vi "ReplaceControlByLabelText.vi"(8 "error in (no error)":errorcluster, 9 "Replacement Path":path, 10 "Control Label.text":string, 11 "VI ref":refnum<vi>) -> (0 "error out":errorcluster, 2 "New Control Ref":refnum<vi>, 3 "VI ref":refnum<vi>)   [LabVIEW 2019, in "BlueUtilityScripts.lvlib"]
uses:
  BlueUtilityScripts.lvlib
  <vilib>/Utility/error.llb/Error Cluster From Error Code.vi
  <vilib>/ErrorRing/Error Ring.xnode
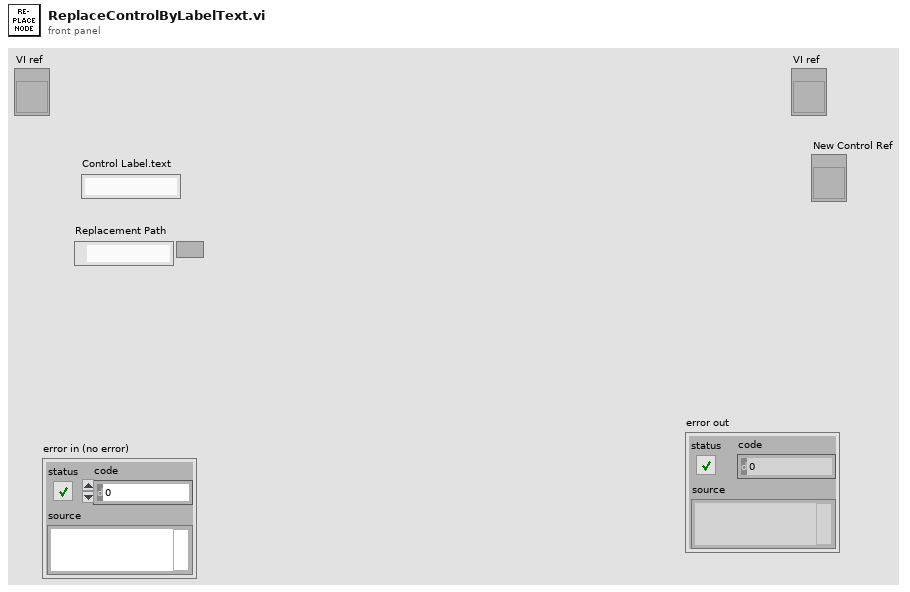
[diagram p1: front panel]
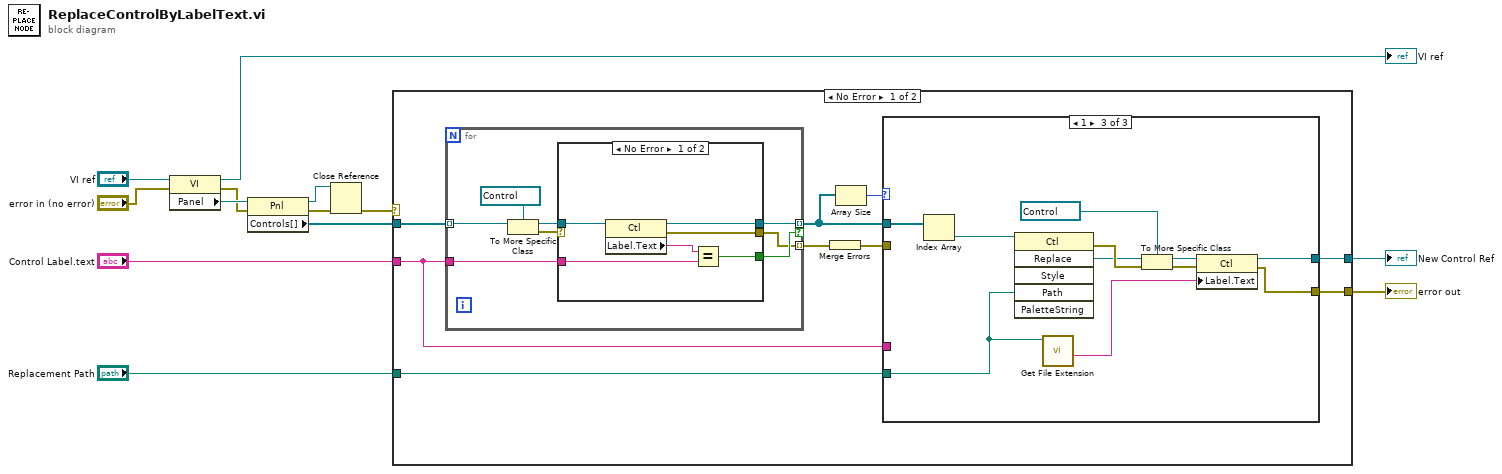
[diagram p0: block diagram]
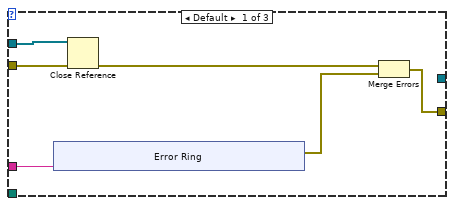
[diagram p2: hidden frame]
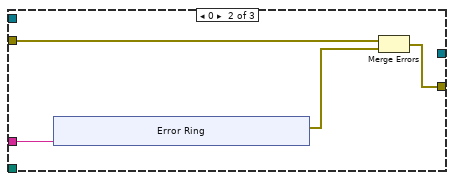
[diagram p3: hidden frame]
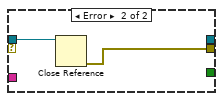
[diagram p4: hidden frame]
diagram:
  n1 = property class="VI"(reference="VI ref", error in="error in (no error)") -> (reference out=→"VI ref":refnum<vi>, error out=w8:errorcluster, "Panel"=w13:refnum<vi>)
  n2 = property class="Pnl"(reference=w13, error in=w8) -> (reference out=w6:refnum<vi>, error out=w7:errorcluster, "Controls[]"=w9:refnum<vi>[])
  n3 = Close Reference(reference=w6, error in (no error)=w7) -> (error out=w5:errorcluster)
  n4 = case shown="No Error" w5 {
    selector: w5 -> [_ w74]
    tunnel: w9 -> [w22 _]
    tunnel: "Control Label.text" -> [w20 _]
    tunnel: "Replacement Path" -> [w16 _]
    tunnel: [w15 w74] -> w1
    tunnel: [w14 _] -> w2
    frame No Error {
      n5 = for {
        tunnel: w22 -> [w65] mode=indexing
        tunnel: [w63] -> w17 mode=indexing if=w59
        tunnel: w20 -> [w60]
        tunnel: [w58] -> w19 mode=indexing
        n6 = To More Specific Class(target class=refnum<vi> refnum ("Other Refnum"), reference=w65) -> (specific class reference=w64:refnum<vi>, error out=w61:errorcluster)  [unwired: 1 in]
        n7 = case shown="No Error" w61 {
          tunnel: w64 -> [w71 w73]
          tunnel: [w70 _] -> w63
          tunnel: w60 -> [w68 _]
          tunnel: [w67 _] -> w59
          tunnel: [w66 w72] -> w58
          frame No Error {
            n8 = property class="Ctl"(reference=w71) -> (reference out=w70:refnum<vi>, error out=w66:errorcluster, "Label.Text"=w69:string)  [unwired: 1 in]
            n9 = Equal?(x=w69, y=w68) -> (x = y?=w67:bool)
          }
          frame Error {
            n10 = Close Reference(reference=w73) -> (error out=w72:errorcluster)  [unwired: 1 in]
          }
        }
      }
      n11 = Merge Errors(w19) -> (w18:errorcluster)
      n12 = Array Size(array=w17) -> (size(s)=w21:i32)
      n13 = case shown="1" w21 {
        tunnel: w20 -> [w28 w39 _]
        tunnel: w18 -> [w24 w38 _]
        tunnel: [w26 w36 w48] -> w15
        tunnel: w17 -> [w25 _ w57]
        tunnel: w16 -> [_ _ w49]
        tunnel: [_ _ w47] -> w14
        frame Default {
          n14 = xnode "Error Ring"("parameter 0"=w28) -> ("error out"=w27:errorcluster)
          n15 = Close Reference(reference=w25, error in (no error)=w24) -> (error out=w23:errorcluster)
          n16 = Merge Errors(w23, w27) -> (w26:errorcluster)
        }
        frame 0 {
          n17 = xnode "Error Ring"("parameter 0"=w39) -> ("error out"=w37:errorcluster)
          n18 = Merge Errors(w38, w37) -> (w36:errorcluster)
        }
        frame 1 {
          n19 = Index Array(array=w57) -> (element=w50:refnum<vi>)  [unwired: 1 in]
          n20 = invoke class="Ctl" method="Replace"(reference=w50, "Path"=w49) -> (error out=w55:errorcluster, "Replace"=w52:refnum<vi>)  [unwired: 4 in, 4 out]
          n21 = call <vilib>:"Get File Extension.vi"("file"=w49) -> ("filename without extension"=w54:string)  [unwired: 6 in, 4 out]
          n22 = To More Specific Class(target class=refnum<vi> refnum ("Other Refnum"), reference=w52, error in=w55) -> (specific class reference=w53:refnum<vi>, error out=w56:errorcluster)
          n23 = property class="Ctl"(reference=w53, error in=w56, "Label.Text"=w54) -> (reference out=w47:refnum<vi>, error out=w48:errorcluster)
        }
      }
    }
    frame Error {
    }
  }
  "error out" <- w1
  "New Control Ref" <- w2
